vi "Read Log file ref.vi"(11 "BuildManager in":refnum<class "BuildManager.lvclass">) -> (2 "Log file ref":refnum<file>, 3 "BuildManager out":refnum<class "BuildManager.lvclass">)   [LabVIEW 2019, in "SolutionBuilder.lvlib" / "BuildManager.lvclass"]
uses:
  BuildManager.lvclass
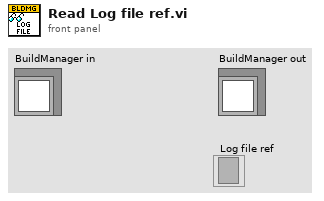
[diagram p1: front panel]
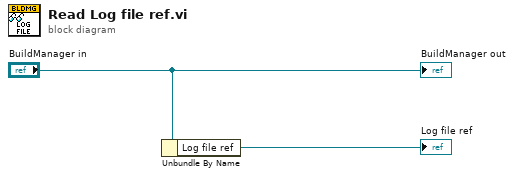
[diagram p0: block diagram]
diagram:
  n1 = Unbundle By Name("BuildManager in") -> ("Log file ref"=→"Log file ref":refnum<file>)
  "BuildManager out" <- "BuildManager in"
